vi "Save Location.vi"(8 "Timer Seconds":dbl, 9 "Counter":dbl, 10 "String":string, 11 "Current":dbl) -> (3 "Saving":bool)   [LabVIEW 2012]
uses:
  <vilib>/Utility/file.llb/Write To Spreadsheet File (string).vi
  <vilib>/Utility/file.llb/Read From Spreadsheet File (string).vi
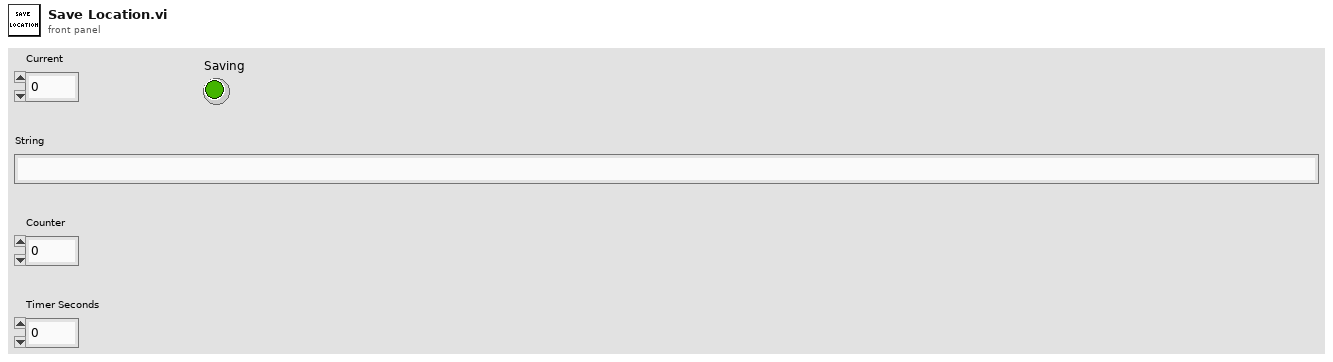
[diagram p1: front panel]
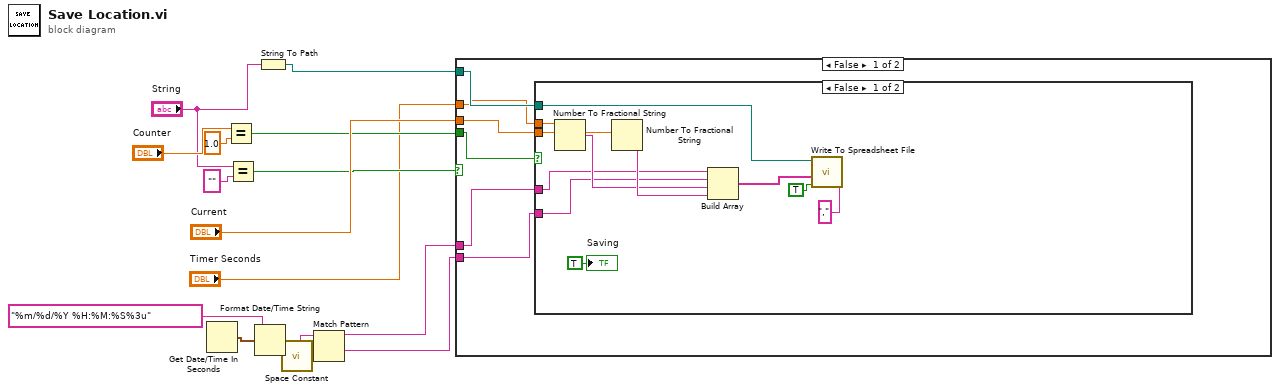
[diagram p0: block diagram]
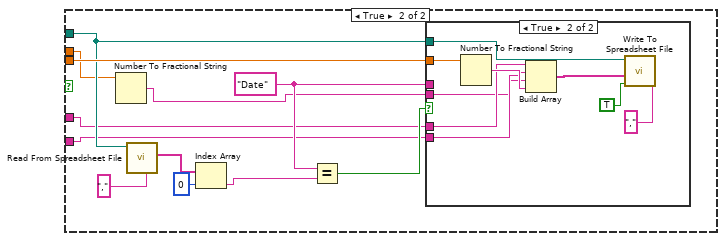
[diagram p2: hidden frame]
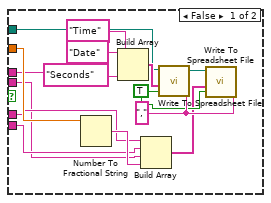
[diagram p3: hidden frame]
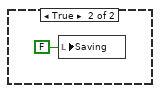
[diagram p4: hidden frame]
diagram:
  n1 = Get Date/Time In Seconds() -> (seconds since 1Jan1904=w4:timestamp)
  n2 = Equal?(x="Counter", y=1.0) -> (x = y?=w8:bool)
  n3 = Equal?(x="String", y="") -> (x = y?=w14:bool)
  n4 = Format Date/Time String(time format string (%c)="%m/%d/%Y %H:%M:%S%3u", seconds (now)=w4) -> (date/time string=w6:string)  [unwired: 1 in]
  n5 = String To Path(string="String") -> (path=w9:path)
  n6 = call <vilib>:"Space Constant.vi"() -> ("String"=w7:string)
  n7 = Match Pattern(string=w6, regular expression=w7) -> (before substring=w2:string, after substring=w1:string)  [unwired: 1 in, 2 out]
  n8 = case shown="False" w14 {
    tunnel: "Current" -> [w21 _]
    tunnel: w8 -> [w20 _]
    tunnel: w9 -> [w19 _]
    tunnel: "Timer Seconds" -> [w18 _]
    tunnel: w2 -> [w17 _]
    tunnel: w1 -> [w16 _]
    frame False {
      n9 = case shown="False" w20 {
        tunnel: w21 -> [w28 w44]
        tunnel: w19 -> [w26 w43]
        tunnel: w18 -> [w25 w35]
        tunnel: w17 -> [w23 w37]
        tunnel: w16 -> [w22 w36]
        frame False {
          n10 = Number To Fractional String(number=w25) -> (F-format string=w24:string)  [unwired: 3 in]
          n11 = Number To Fractional String(number=w28) -> (F-format string=w29:string)  [unwired: 3 in]
          n12 = Build Array(w23, w22, w24, w29) -> (w32:string[])
          n13 = call-poly <vilib>:"Write To Spreadsheet File.vi"("delimiter (\\t)"="," ("delimiter (\\t)"), "append to file? (new file:F)"=TRUE, "1D data"=w32, "file path (dialog if empty)"=w26) -> ()  [unwired: 4 in, 1 out]
          "Saving" <- TRUE
        }
        frame True {
          w39 = "Date" ("element")
          n14 = Number To Fractional String(number=w35) -> (F-format string=w34:string)  [unwired: 3 in]
          n15 = call-poly <vilib>:"Read From Spreadsheet File.vi"("delimiter (\\t)"="," ("delimiter (\\t)"), "file path (dialog if empty)"=w43) -> ("first row"=w42:string[])  [unwired: 5 in, 4 out]
          n16 = Index Array(array=w42, index=0) -> (element=w40:string)
          n17 = Equal?(x=w39, y=w40) -> (x = y?=w38:bool)
          n18 = case shown="True" w38 {
            tunnel: w44 -> [w58 w66]
            tunnel: w43 -> [w52 w63]
            tunnel: w39 -> [w51 _]
            tunnel: w37 -> [w47 w62]
            tunnel: w36 -> [w46 w61]
            tunnel: w34 -> [w45 w60]
            frame False {
              w57 = "," ("delimiter (\\t)")
              w56 = TRUE ("append to file? (new file:F)")
              n19 = Number To Fractional String(number=w58) -> (F-format string=w55:string)  [unwired: 3 in]
              n20 = Build Array("Date" ("element"), "Time" ("element"), "Seconds" ("element"), w51) -> (w59:string[])
              n21 = Build Array(w47, w46, w45, w55) -> (w54:string[])
              n22 = call-poly <vilib>:"Write To Spreadsheet File.vi"("delimiter (\\t)"=w57, "append to file? (new file:F)"=w56, "1D data"=w59, "file path (dialog if empty)"=w52) -> ("new file path (Not A Path if cancelled)"=w53:path)  [unwired: 4 in]
              n23 = call-poly <vilib>:"Write To Spreadsheet File.vi"("delimiter (\\t)"=w57, "append to file? (new file:F)"=w56, "1D data"=w54, "file path (dialog if empty)"=w53) -> ()  [unwired: 4 in, 1 out]
            }
            frame True {
              n24 = Number To Fractional String(number=w66) -> (F-format string=w65:string)  [unwired: 3 in]
              n25 = Build Array(w62, w61, w60, w65) -> (w64:string[])
              n26 = call-poly <vilib>:"Write To Spreadsheet File.vi"("delimiter (\\t)"="," ("delimiter (\\t)"), "append to file? (new file:F)"=TRUE, "1D data"=w64, "file path (dialog if empty)"=w63) -> ()  [unwired: 4 in, 1 out]
            }
          }
        }
      }
    }
    frame True {
      n27 = local write "Saving"(FALSE ("Saving")) -> ()
    }
  }
